vi "PUT-FILE.vi"(0 "client handle":T4, 1 "output file":path=path "", 2 "Error code options":T1={"1xx (info)"=FALSE, "2xx (success)"=FALSE, "3xx (redirect)"=FALSE, "4xx (client error)"=TRUE, "5xx (server error)"=TRUE, "Other"=TRUE}, 3 "BlueLogParent in":refnum<class "BlueLogParent_OpenSource.lvclass">, 5 "url":string, 7 "file":path, 11 "error in (no error)":errorcluster, 12 "timeout (10000)":i32=10000) -> (4 "client handle out":T4, 6 "headers":T3[](array[typedef]), 8 "body":string, 10 "HTTP response code":T2, 15 "error out":errorcluster)   [LabVIEW 2020, in "Blue Easy HTTP OpenSource.lvlib"]
doc: "Sends a Web request that submits data or a file to a server, Web page, or Web service. This VI uses the PUT HTTP method. Refer to the World Wide Web Consortium Web site at www.w3.org for more information about HTTP method definitions, including the PUT method.\n\nYou can assign a client handle to add authentication credentials, HTTP headers, or a cookie to Web requests made by the PUT VI. Use the OpenHandle VI to open a client handle and establish credentials. Use the AddHeader VI to add header lines to Web requests made by the PUT VI."
uses:
  Blue Easy HTTP OpenSource.lvlib
  <vilib>/httpClient/ClientHandle.ctl
  HTTP Header.ctl
  HTTP response code.ctl
  HTTP error on codes.ctl
  <userlib>/Blue Origin/BlueLogParent_OpenSource/BlueLogParentClass/BlueLogParent_OpenSource.lvclass
  Interpret Header.vi
  <vilib>/dlg_ctls.llb/Space Constant.vi
  <vilib>/Utility/error.llb/Trim Whitespace.vi
  <vilib>/Utility/error.llb/Error Cluster From Error Code.vi
  <vilib>/httpClient/LabVIEWHTTPClient.lvlib
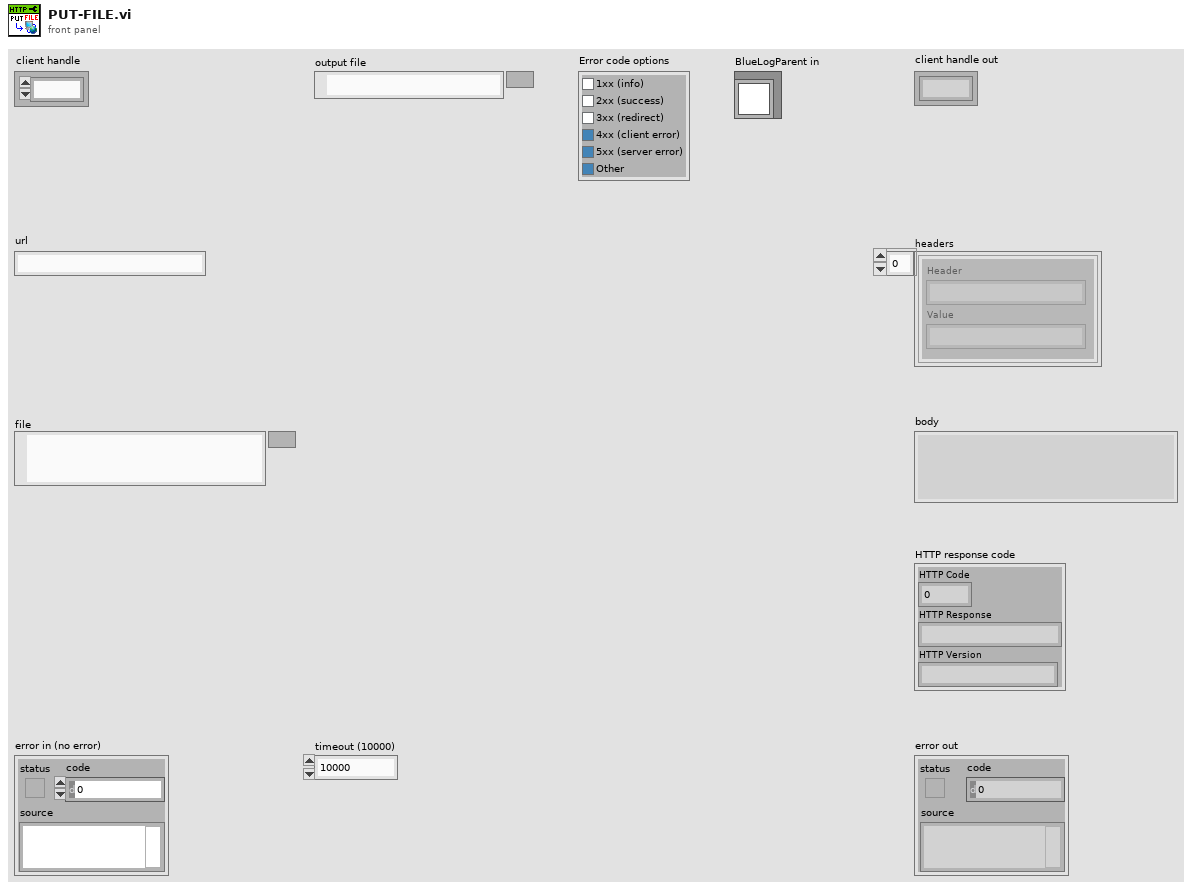
[diagram p1: front panel]
types:
  T1 = typedef "Blue Easy HTTP OpenSource.lvlib/HTTP error on codes.ctl" = cluster{"1xx (info)":bool, "2xx (success)":bool, "3xx (redirect)":bool, "4xx (client error)":bool, "5xx (server error)":bool, "Other":bool}
  T2 = typedef "Blue Easy HTTP OpenSource.lvlib/HTTP response code.ctl" = cluster{"HTTP Code":u16, "HTTP Response":string, "HTTP Version":string}
  T3 = typedef "Blue Easy HTTP OpenSource.lvlib/HTTP Header.ctl" = cluster{"Header":string, "Value":string}
  T4 = typedef "LabVIEWHTTPClient.lvlib/ClientHandle.ctl" = refnum<k1>
  T5 = typedef "BlueLogParent_OpenSource.lvclass/BlueLogParentLevel.ctl" = enum16{"DEBUG", "INFO", "WARNING", "ERROR", "CRITICAL"}
  T6 = typedef "BlueLogParent_OpenSource.lvclass/BlueLogParentOptions.ctl" = cluster{"timestamp (now)":dbl, "Call chain (here)":string, "Count (1)":u16, "Font (override)":T7, "Add row separator? (T)":bool}
  T7 = typedef "BlueLogParent_OpenSource.lvclass/BlueLogParentFont.ctl" = cluster{"Font Name":string, "Size":u16, "Bold":bool, "Italic":bool, "Underline":bool, "Strikeout":bool, "Color":u32}
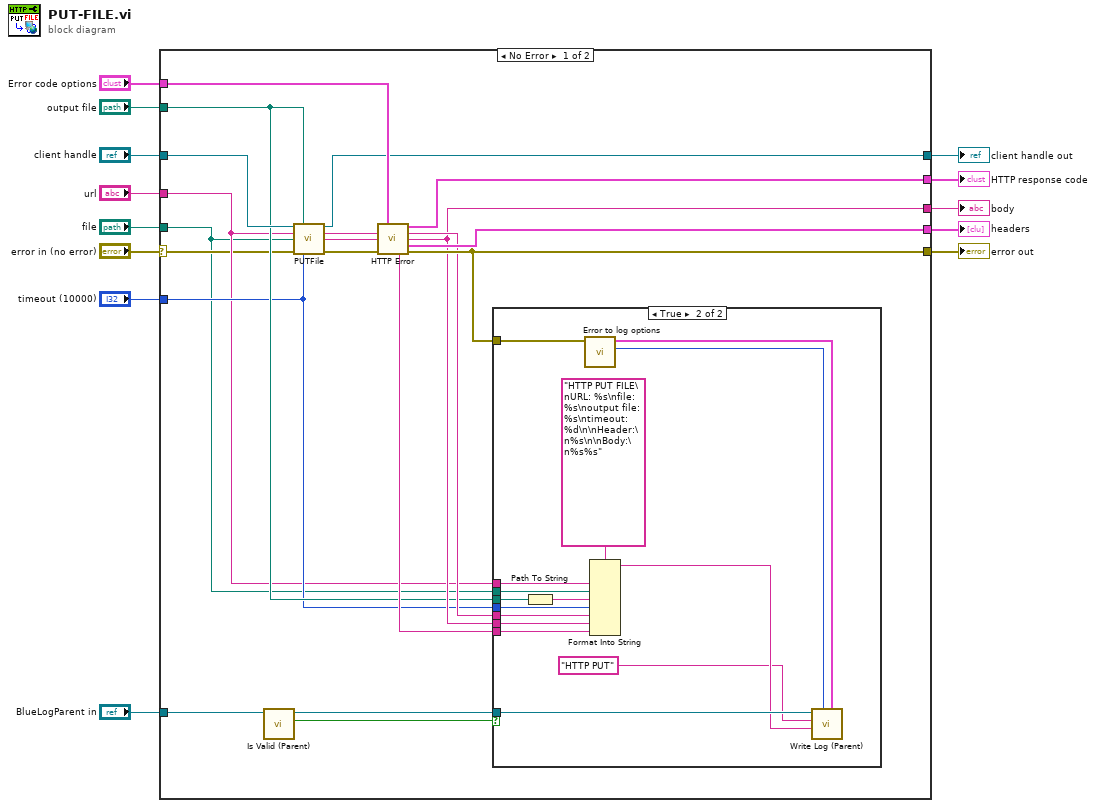
[diagram p0: block diagram]
diagram:
  n1 = case shown="No Error" "error in (no error)" {
    selector: "error in (no error)" -> [w15 w50]
    tunnel: [w31 w50] -> w13
    tunnel: "file" -> [w14 _]
    tunnel: "timeout (10000)" -> [w20 _]
    tunnel: "url" -> [w19 _]
    tunnel: "output file" -> [w22 _]
    tunnel: "client handle" -> [w23 w49]
    tunnel: [w21 w49] -> w6
    tunnel: [w33 _] -> w5
    tunnel: [w25 _] -> w4
    tunnel: [w32 _] -> w3
    tunnel: "Error code options" -> [w30 _]
    tunnel: "BlueLogParent in" -> [w29 _]
    frame No Error {
      n2 = call-dynamic "Is Valid (Parent).vi"("BlueLogParent in"=w29) -> ("Is Valid?"=w28:bool, "BlueLogParent out"=w27:refnum<class "BlueLogParent_OpenSource.lvclass">)  [unwired: 8 in, 1 out]
      n3 = call <vilib>:"PUTFile.vi"("client handle"=w23, "output file"=w22, "url"=w19, "file"=w14, "error in (no error)"=w15, "timeout (10000)"=w20) -> ("client handle out"=w21:T4, "headers"=w18:string, "body"=w17:string, "error out"=w16:errorcluster)  [unwired: 6 in]
      n4 = call "HTTP Error.vi"("Error code options"=w30, "Header"=w18, "body"=w17, "error in (no error)"=w16) -> ("HTTP response code"=w32:T2, "Header (dup)"=w26:string, "body (dup)"=w25:string, "Header Values"=w33:T3[], "Error log"=w24:string, "error out"=w31:errorcluster)  [unwired: 6 in]
      n5 = case shown="True" w28 {
        tunnel: w31 -> [_ w39]
        tunnel: w19 -> [_ w47]
        tunnel: w22 -> [_ w46]
        tunnel: w14 -> [_ w45]
        tunnel: w20 -> [_ w43]
        tunnel: w26 -> [_ w42]
        tunnel: w25 -> [_ w41]
        tunnel: w27 -> [_ w40]
        tunnel: w24 -> [_ w34]
        frame False {
        }
        frame True {
          n6 = Path To String(path=w46) -> (string=w44:string)
          n7 = call "Error to log options.vi"("error in (no error)"=w39) -> ("Logging level"=w37:T5, "Options"=w38:T6)  [unwired: 9 in]
          n8 = Format Into String(format string="HTTP PUT FILE\nURL: %s\nfile: %s\noutput file: %s\ntimeout: %d\n\nHeader:\n%s\n\nBody:\n%s%s", w47, w45, w44, w43, w42, w41, w34) -> (resulting string=w36:string)  [unwired: 2 in, 1 out]
          n9 = call-dynamic "Write Log (Parent).vi"("Options"=w38, "Logging level (INFO)"=w37, "Message"=w36, "Message Title"="HTTP PUT" ("Unique ID"), "BlueLogParent in"=w40) -> ()  [unwired: 5 in, 2 out]
        }
      }
    }
    frame Error {
    }
  }
  "error out" <- w13
  "client handle out" <- w6
  "body" <- w4
  "headers" <- w5
  "HTTP response code" <- w3
